vi "Global 1.vi"() -> ()   [LabVIEW 2024, in "Launcher_DTU.lvlib"]
uses:
  Launcher_DTU.lvlib
panel:
  out "N58 Done":bool
  out "N582":bool
  out "N581":bool
  out "ENG_Mode":bool
  out "Bar_init_2":bool
  out "Bar_init_1":bool
  in  "Barcode_2":string
  in  "Barcode_1":string
  out "Exit":bool
  out "PS":bool
  out "DAQ2":bool
  out "DAQ1":bool
  out "PCAN2":bool
  out "PCAN1":bool
  out "Write_Exit 2":bool
  out "Write_Exit":bool
  in  "Selected Config":string
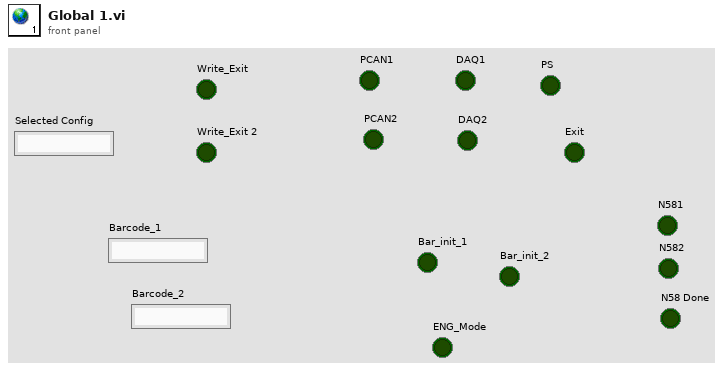
[diagram p1: front panel]
diagram:
